vi "Coords.vi"(10 "Data Points":dbl[][](array[numeric])) -> (0 "Reflectivity Vector":dbl[](array[numeric]), 1 "Y Vector":dbl[](array[numeric]), 4 "Z Vector":dbl[](array[numeric]), 5 "X Vector":dbl[](array[numeric]))   [LabVIEW 2017]
panel:
  out "theta":dbl
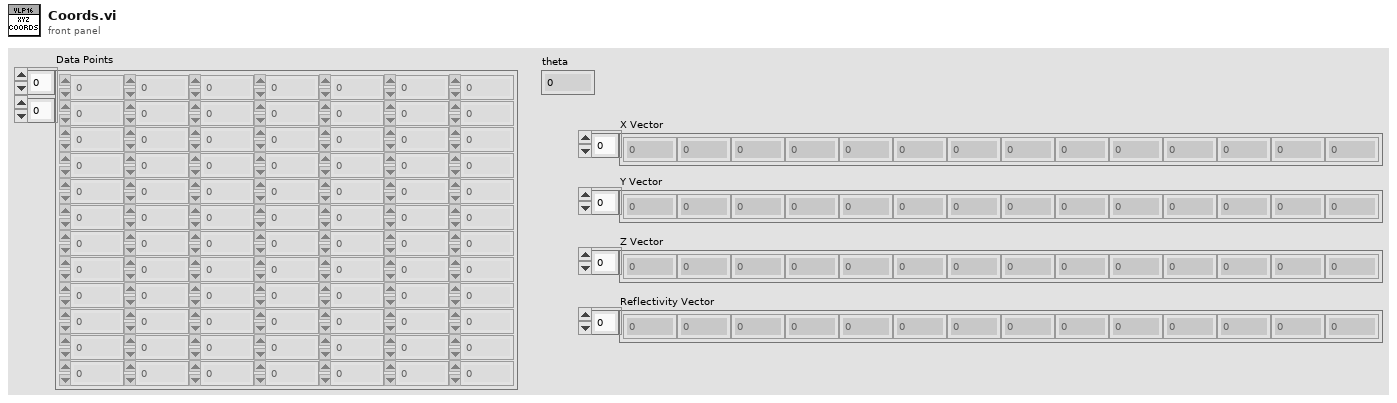
[diagram p1: front panel]
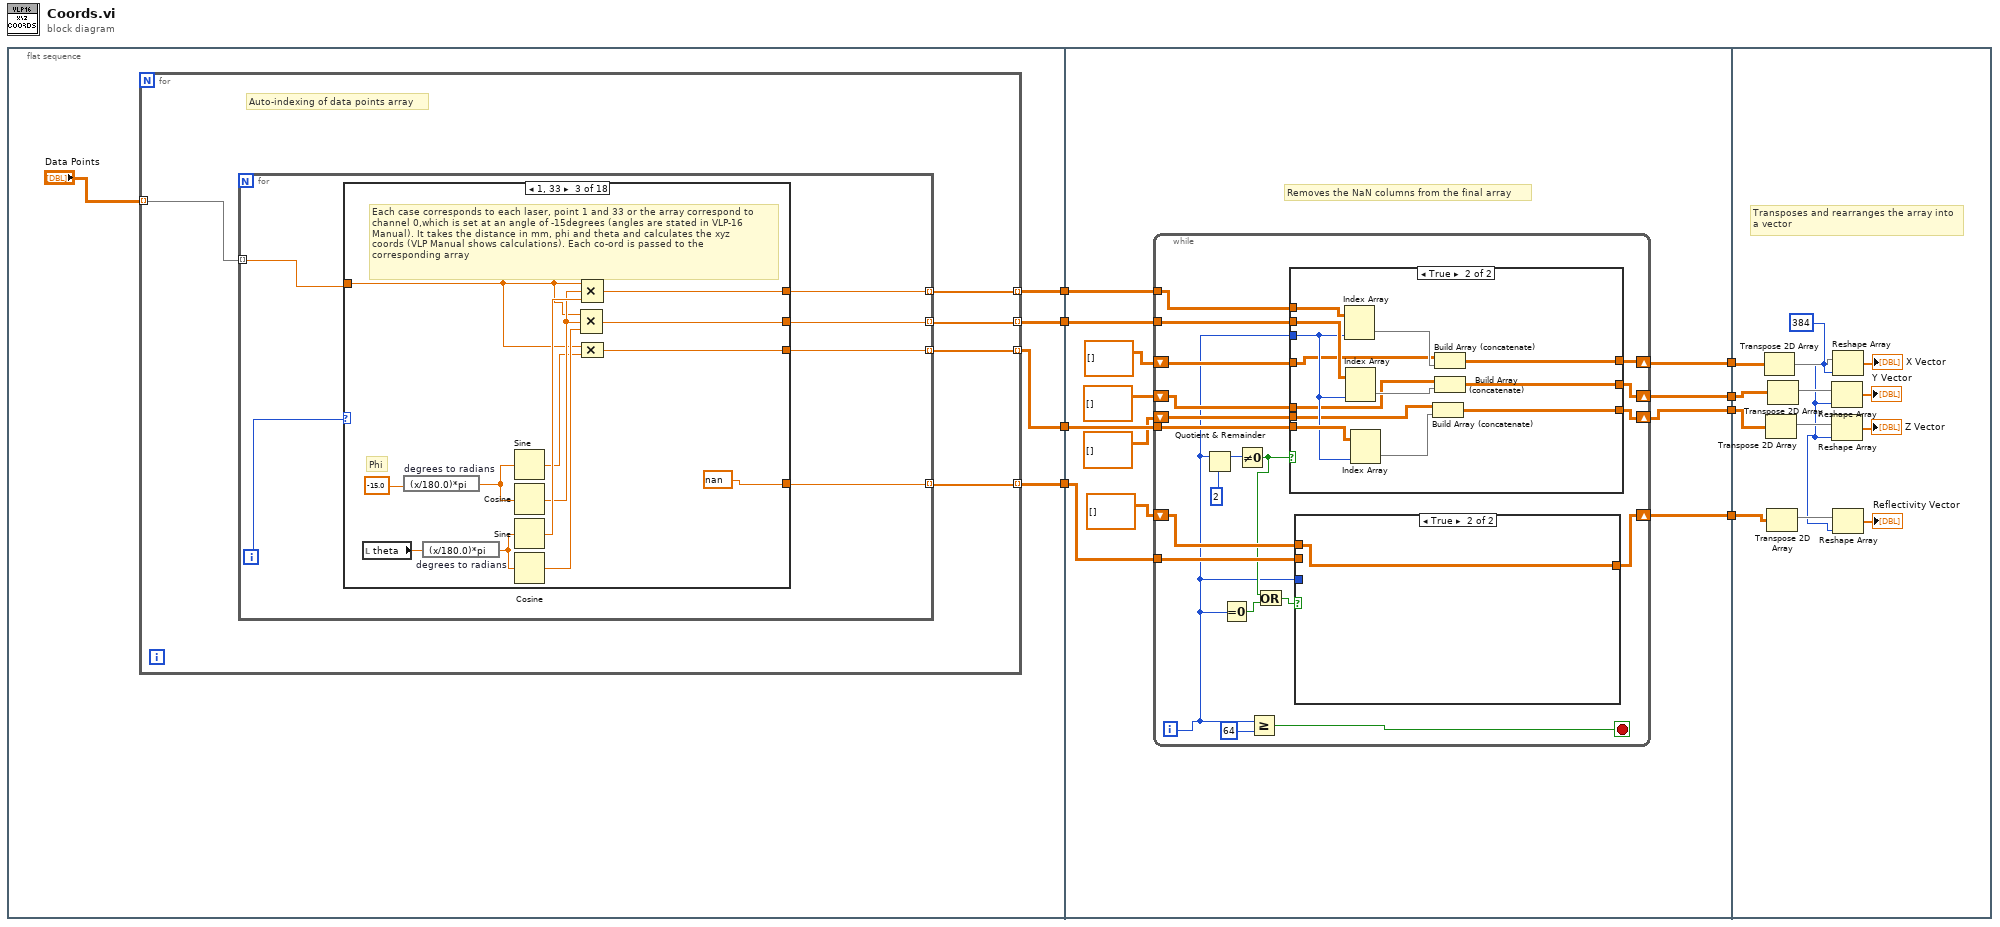
[diagram p0: block diagram]
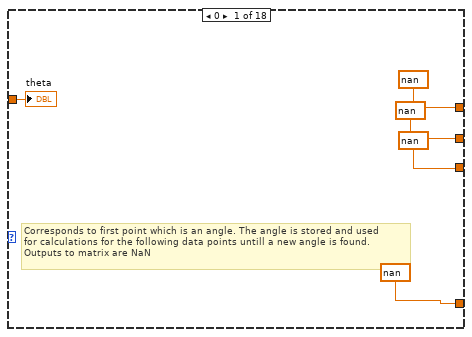
[diagram p2: hidden frame]
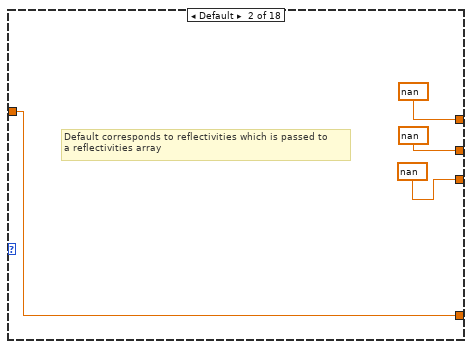
[diagram p3: hidden frame]
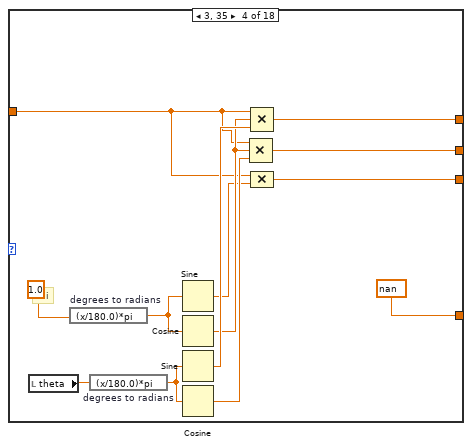
[diagram p4: hidden frame]
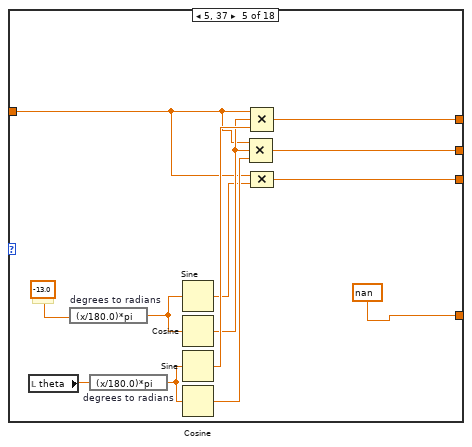
[diagram p5: hidden frame]
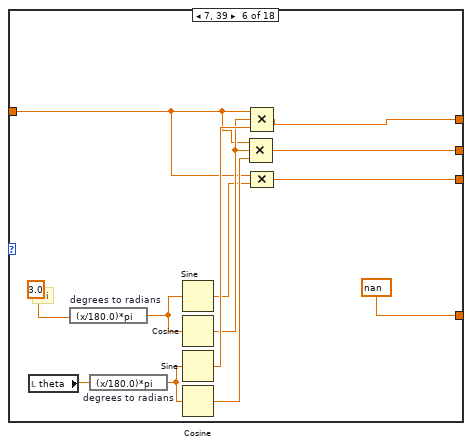
[diagram p6: hidden frame]
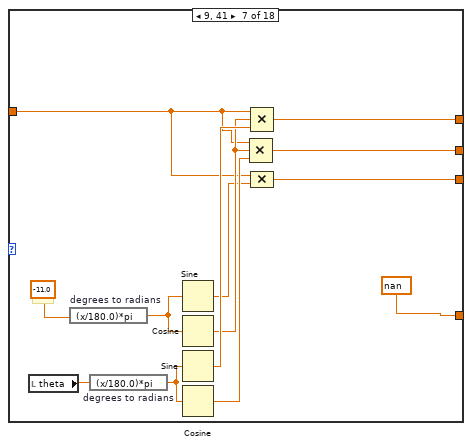
[diagram p7: hidden frame]
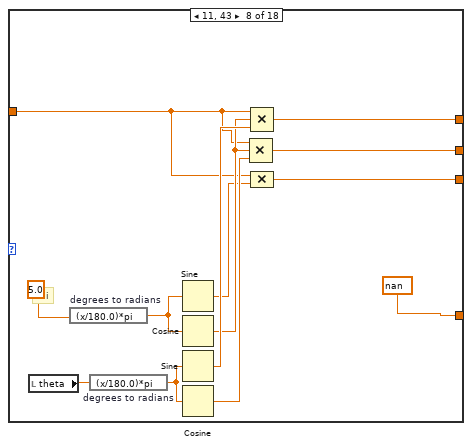
[diagram p8: hidden frame]
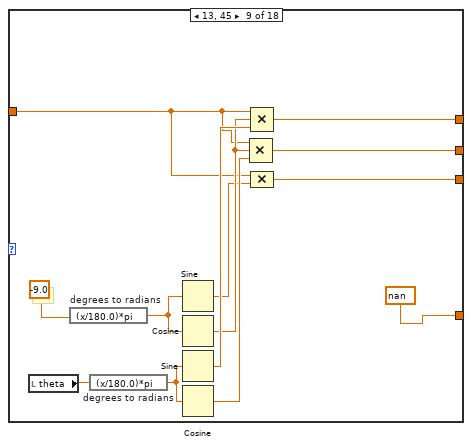
[diagram p9: hidden frame]
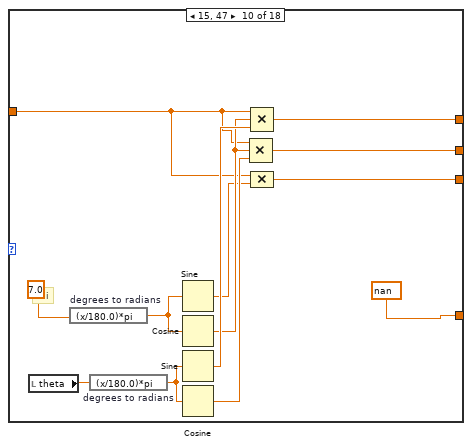
[diagram p10: hidden frame]
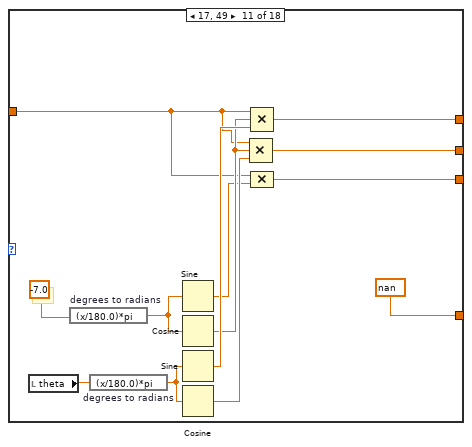
[diagram p11: hidden frame]
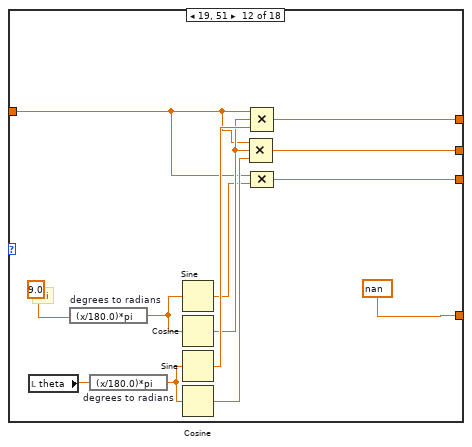
[diagram p12: hidden frame]
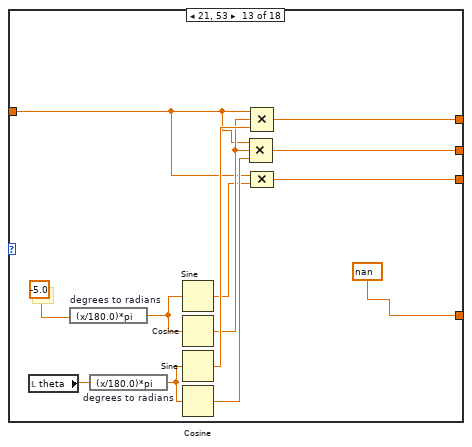
[diagram p13: hidden frame]
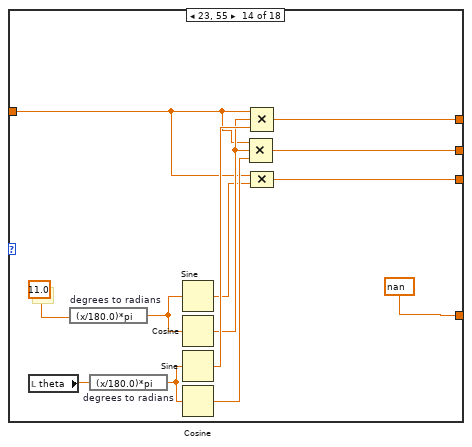
[diagram p14: hidden frame]
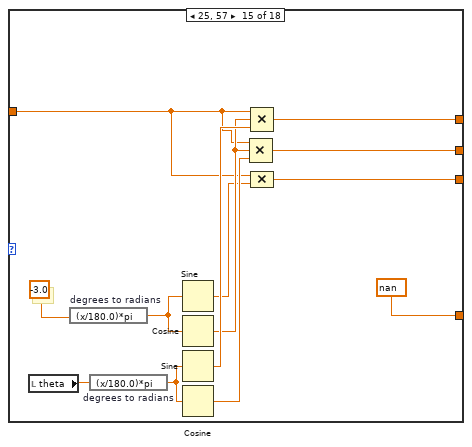
[diagram p15: hidden frame]
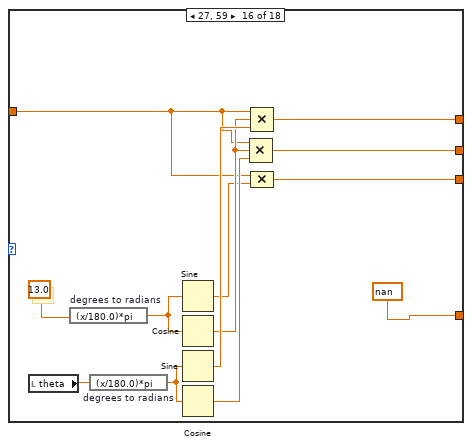
[diagram p16: hidden frame]
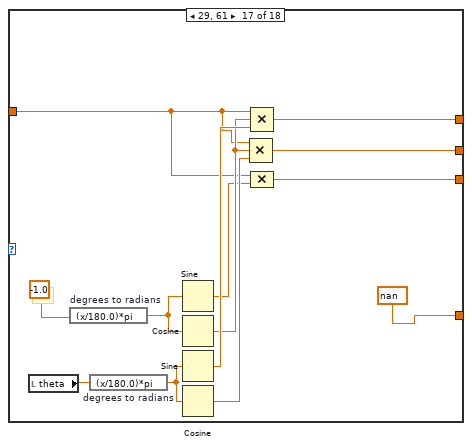
[diagram p17: hidden frame]
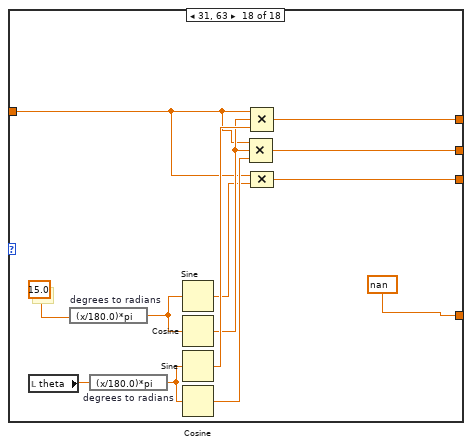
[diagram p18: hidden frame]
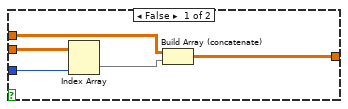
[diagram p19: hidden frame]
diagram:
  n1 = flat-sequence {
    tunnel: [w12] -> w8
    tunnel: [w11] -> w7
    tunnel: [w10] -> w6
    tunnel: [w9] -> w2
    tunnel: w8 -> [w253]
    tunnel: w7 -> [w252]
    tunnel: w6 -> [w251]
    tunnel: [w249] -> w5
    tunnel: [w246] -> w4
    tunnel: [w245] -> w3
    tunnel: w2 -> [w243]
    tunnel: [w242] -> w1
    tunnel: w5 -> [w306]
    tunnel: w4 -> [w307]
    tunnel: w3 -> [w308]
    tunnel: w1 -> [w298]
    frame #0 {
      n2 = for {
        tunnel: "Data Points" -> [w18] mode=indexing
        tunnel: [w17] -> w12 mode=indexing
        tunnel: [w16] -> w11 mode=indexing
        tunnel: [w15] -> w10 mode=indexing
        tunnel: [w14] -> w9 mode=indexing
        # "Auto-indexing of data points array"
        n3 = for {
          tunnel: w18 -> [w23] mode=indexing
          tunnel: [w22] -> w17 mode=indexing
          tunnel: [w21] -> w16 mode=indexing
          tunnel: [w20] -> w15 mode=indexing
          tunnel: [w19] -> w14 mode=indexing
          i -> [w24]
          n4 = case shown="1, 33" w24 {
            tunnel: w23 -> [w29 w30 w43 w56 w69 w82 w95 w108 w121 w134 w147 w160 w173 w186 w199 w212 w225 w238]
            tunnel: [nan nan w37 w50 w63 w76 w89 w102 w115 w128 w141 w154 w167 w180 w193 w206 w219 w232] -> w22
            tunnel: [nan nan w36 w49 w62 w75 w88 w101 w114 w127 w140 w153 w166 w179 w192 w205 w218 w231] -> w21
            tunnel: [nan nan w35 w48 w61 w74 w87 w100 w113 w126 w139 w152 w165 w178 w191 w204 w217 w230] -> w20
            tunnel: [nan w30 nan nan nan nan nan nan nan nan nan nan nan nan nan nan nan nan] -> w19
            frame 0 {
              # "Corresponds to first point which is an angle. The angle is stored and used\nfor calculations for the following data points untill a new angle is found.\nOutputs to matrix are NaN"
              "theta" <- w29
            }
            frame Default {
              # "Default corresponds to reflectivities which is passed to\na reflectivities array"
            }
            frame 1, 33 {
              # "Each case corresponds to each laser, point 1 and 33 or the array correspond to \nchannel 0,which is set at an angle of -15degrees (angles are stated in VLP-16 \nManual). It takes the distance in mm, phi and theta and calculates the xyz \ncoords (VLP Manual shows calculations). Each co-ord is passed to the \ncorresponding array"
              # "Phi"
              n5 = local read "theta"() -> (w38:dbl)
              n6 = expression code="(x/180.0)*pi" "degrees to radians"(-15.0) -> (w40:dbl)
              n7 = expression code="(x/180.0)*pi" "degrees to radians"(w38) -> (w39:dbl)
              n8 = Sine(x=w40) -> (sin(x)=w42:dbl)
              n9 = Cosine(x=w40) -> (cos(x)=w45:dbl)
              n10 = Sine(x=w39) -> (sin(x)=w46:dbl)
              n11 = Cosine(x=w39) -> (cos(x)=w44:dbl)
              n12 = Compound Arithmetic op=MULTIPLY(w43, w45, w44) -> (w36:dbl)
              n13 = Compound Arithmetic op=MULTIPLY(w43, w45, w46) -> (w37:dbl)
              n14 = Compound Arithmetic op=MULTIPLY(w43, w42) -> (w35:dbl)
            }
            frame 3, 35 {
              # "Phi"
              n15 = local read "theta"() -> (w51:dbl)
              n16 = expression code="(x/180.0)*pi" "degrees to radians"(1.0) -> (w53:dbl)
              n17 = expression code="(x/180.0)*pi" "degrees to radians"(w51) -> (w52:dbl)
              n18 = Sine(x=w53) -> (sin(x)=w55:dbl)
              n19 = Cosine(x=w53) -> (cos(x)=w58:dbl)
              n20 = Sine(x=w52) -> (sin(x)=w59:dbl)
              n21 = Cosine(x=w52) -> (cos(x)=w57:dbl)
              n22 = Compound Arithmetic op=MULTIPLY(w56, w58, w57) -> (w49:dbl)
              n23 = Compound Arithmetic op=MULTIPLY(w56, w58, w59) -> (w50:dbl)
              n24 = Compound Arithmetic op=MULTIPLY(w56, w55) -> (w48:dbl)
            }
            frame 5, 37 {
              # "Phi"
              n25 = local read "theta"() -> (w64:dbl)
              n26 = expression code="(x/180.0)*pi" "degrees to radians"(-13.0) -> (w66:dbl)
              n27 = expression code="(x/180.0)*pi" "degrees to radians"(w64) -> (w65:dbl)
              n28 = Sine(x=w66) -> (sin(x)=w68:dbl)
              n29 = Cosine(x=w66) -> (cos(x)=w71:dbl)
              n30 = Sine(x=w65) -> (sin(x)=w72:dbl)
              n31 = Cosine(x=w65) -> (cos(x)=w70:dbl)
              n32 = Compound Arithmetic op=MULTIPLY(w69, w71, w70) -> (w62:dbl)
              n33 = Compound Arithmetic op=MULTIPLY(w69, w71, w72) -> (w63:dbl)
              n34 = Compound Arithmetic op=MULTIPLY(w69, w68) -> (w61:dbl)
            }
            frame 7, 39 {
              # "Phi"
              n35 = local read "theta"() -> (w77:dbl)
              n36 = expression code="(x/180.0)*pi" "degrees to radians"(3.0) -> (w79:dbl)
              n37 = expression code="(x/180.0)*pi" "degrees to radians"(w77) -> (w78:dbl)
              n38 = Sine(x=w79) -> (sin(x)=w81:dbl)
              n39 = Cosine(x=w79) -> (cos(x)=w84:dbl)
              n40 = Sine(x=w78) -> (sin(x)=w85:dbl)
              n41 = Cosine(x=w78) -> (cos(x)=w83:dbl)
              n42 = Compound Arithmetic op=MULTIPLY(w82, w84, w83) -> (w75:dbl)
              n43 = Compound Arithmetic op=MULTIPLY(w82, w84, w85) -> (w76:dbl)
              n44 = Compound Arithmetic op=MULTIPLY(w82, w81) -> (w74:dbl)
            }
            frame 9, 41 {
              # "Phi"
              n45 = local read "theta"() -> (w90:dbl)
              n46 = expression code="(x/180.0)*pi" "degrees to radians"(-11.0) -> (w92:dbl)
              n47 = expression code="(x/180.0)*pi" "degrees to radians"(w90) -> (w91:dbl)
              n48 = Sine(x=w92) -> (sin(x)=w94:dbl)
              n49 = Cosine(x=w92) -> (cos(x)=w97:dbl)
              n50 = Sine(x=w91) -> (sin(x)=w98:dbl)
              n51 = Cosine(x=w91) -> (cos(x)=w96:dbl)
              n52 = Compound Arithmetic op=MULTIPLY(w95, w97, w96) -> (w88:dbl)
              n53 = Compound Arithmetic op=MULTIPLY(w95, w97, w98) -> (w89:dbl)
              n54 = Compound Arithmetic op=MULTIPLY(w95, w94) -> (w87:dbl)
            }
            frame 11, 43 {
              # "Phi"
              n55 = local read "theta"() -> (w103:dbl)
              n56 = expression code="(x/180.0)*pi" "degrees to radians"(5.0) -> (w105:dbl)
              n57 = expression code="(x/180.0)*pi" "degrees to radians"(w103) -> (w104:dbl)
              n58 = Sine(x=w105) -> (sin(x)=w107:dbl)
              n59 = Cosine(x=w105) -> (cos(x)=w110:dbl)
              n60 = Sine(x=w104) -> (sin(x)=w111:dbl)
              n61 = Cosine(x=w104) -> (cos(x)=w109:dbl)
              n62 = Compound Arithmetic op=MULTIPLY(w108, w110, w109) -> (w101:dbl)
              n63 = Compound Arithmetic op=MULTIPLY(w108, w110, w111) -> (w102:dbl)
              n64 = Compound Arithmetic op=MULTIPLY(w108, w107) -> (w100:dbl)
            }
            frame 13, 45 {
              # "Phi"
              n65 = local read "theta"() -> (w116:dbl)
              n66 = expression code="(x/180.0)*pi" "degrees to radians"(-9.0) -> (w118:dbl)
              n67 = expression code="(x/180.0)*pi" "degrees to radians"(w116) -> (w117:dbl)
              n68 = Sine(x=w118) -> (sin(x)=w120:dbl)
              n69 = Cosine(x=w118) -> (cos(x)=w123:dbl)
              n70 = Sine(x=w117) -> (sin(x)=w124:dbl)
              n71 = Cosine(x=w117) -> (cos(x)=w122:dbl)
              n72 = Compound Arithmetic op=MULTIPLY(w121, w123, w122) -> (w114:dbl)
              n73 = Compound Arithmetic op=MULTIPLY(w121, w123, w124) -> (w115:dbl)
              n74 = Compound Arithmetic op=MULTIPLY(w121, w120) -> (w113:dbl)
            }
            frame 15, 47 {
              # "Phi"
              n75 = local read "theta"() -> (w129:dbl)
              n76 = expression code="(x/180.0)*pi" "degrees to radians"(7.0) -> (w131:dbl)
              n77 = expression code="(x/180.0)*pi" "degrees to radians"(w129) -> (w130:dbl)
              n78 = Sine(x=w131) -> (sin(x)=w133:dbl)
              n79 = Cosine(x=w131) -> (cos(x)=w136:dbl)
              n80 = Sine(x=w130) -> (sin(x)=w137:dbl)
              n81 = Cosine(x=w130) -> (cos(x)=w135:dbl)
              n82 = Compound Arithmetic op=MULTIPLY(w134, w136, w135) -> (w127:dbl)
              n83 = Compound Arithmetic op=MULTIPLY(w134, w136, w137) -> (w128:dbl)
              n84 = Compound Arithmetic op=MULTIPLY(w134, w133) -> (w126:dbl)
            }
            frame 17, 49 {
              # "Phi"
              n85 = local read "theta"() -> (w142:dbl)
              n86 = expression code="(x/180.0)*pi" "degrees to radians"(-7.0) -> (w144:dbl)
              n87 = expression code="(x/180.0)*pi" "degrees to radians"(w142) -> (w143:dbl)
              n88 = Sine(x=w144) -> (sin(x)=w146:dbl)
              n89 = Cosine(x=w144) -> (cos(x)=w149:dbl)
              n90 = Sine(x=w143) -> (sin(x)=w150:dbl)
              n91 = Cosine(x=w143) -> (cos(x)=w148:dbl)
              n92 = Compound Arithmetic op=MULTIPLY(w147, w149, w148) -> (w140:dbl)
              n93 = Compound Arithmetic op=MULTIPLY(w147, w149, w150) -> (w141:dbl)
              n94 = Compound Arithmetic op=MULTIPLY(w147, w146) -> (w139:dbl)
            }
            frame 19, 51 {
              # "Phi"
              n95 = local read "theta"() -> (w155:dbl)
              n96 = expression code="(x/180.0)*pi" "degrees to radians"(9.0) -> (w157:dbl)
              n97 = expression code="(x/180.0)*pi" "degrees to radians"(w155) -> (w156:dbl)
              n98 = Sine(x=w157) -> (sin(x)=w159:dbl)
              n99 = Cosine(x=w157) -> (cos(x)=w162:dbl)
              n100 = Sine(x=w156) -> (sin(x)=w163:dbl)
              n101 = Cosine(x=w156) -> (cos(x)=w161:dbl)
              n102 = Compound Arithmetic op=MULTIPLY(w160, w162, w161) -> (w153:dbl)
              n103 = Compound Arithmetic op=MULTIPLY(w160, w162, w163) -> (w154:dbl)
              n104 = Compound Arithmetic op=MULTIPLY(w160, w159) -> (w152:dbl)
            }
            frame 21, 53 {
              # "Phi"
              n105 = local read "theta"() -> (w168:dbl)
              n106 = expression code="(x/180.0)*pi" "degrees to radians"(-5.0) -> (w170:dbl)
              n107 = expression code="(x/180.0)*pi" "degrees to radians"(w168) -> (w169:dbl)
              n108 = Sine(x=w170) -> (sin(x)=w172:dbl)
              n109 = Cosine(x=w170) -> (cos(x)=w175:dbl)
              n110 = Sine(x=w169) -> (sin(x)=w176:dbl)
              n111 = Cosine(x=w169) -> (cos(x)=w174:dbl)
              n112 = Compound Arithmetic op=MULTIPLY(w173, w175, w174) -> (w166:dbl)
              n113 = Compound Arithmetic op=MULTIPLY(w173, w175, w176) -> (w167:dbl)
              n114 = Compound Arithmetic op=MULTIPLY(w173, w172) -> (w165:dbl)
            }
            frame 23, 55 {
              # "Phi"
              n115 = local read "theta"() -> (w181:dbl)
              n116 = expression code="(x/180.0)*pi" "degrees to radians"(11.0) -> (w183:dbl)
              n117 = expression code="(x/180.0)*pi" "degrees to radians"(w181) -> (w182:dbl)
              n118 = Sine(x=w183) -> (sin(x)=w185:dbl)
              n119 = Cosine(x=w183) -> (cos(x)=w188:dbl)
              n120 = Sine(x=w182) -> (sin(x)=w189:dbl)
              n121 = Cosine(x=w182) -> (cos(x)=w187:dbl)
              n122 = Compound Arithmetic op=MULTIPLY(w186, w188, w187) -> (w179:dbl)
              n123 = Compound Arithmetic op=MULTIPLY(w186, w188, w189) -> (w180:dbl)
              n124 = Compound Arithmetic op=MULTIPLY(w186, w185) -> (w178:dbl)
            }
            frame 25, 57 {
              # "Phi"
              n125 = local read "theta"() -> (w194:dbl)
              n126 = expression code="(x/180.0)*pi" "degrees to radians"(-3.0) -> (w196:dbl)
              n127 = expression code="(x/180.0)*pi" "degrees to radians"(w194) -> (w195:dbl)
              n128 = Sine(x=w196) -> (sin(x)=w198:dbl)
              n129 = Cosine(x=w196) -> (cos(x)=w201:dbl)
              n130 = Sine(x=w195) -> (sin(x)=w202:dbl)
              n131 = Cosine(x=w195) -> (cos(x)=w200:dbl)
              n132 = Compound Arithmetic op=MULTIPLY(w199, w201, w200) -> (w192:dbl)
              n133 = Compound Arithmetic op=MULTIPLY(w199, w201, w202) -> (w193:dbl)
              n134 = Compound Arithmetic op=MULTIPLY(w199, w198) -> (w191:dbl)
            }
            frame 27, 59 {
              # "Phi"
              n135 = local read "theta"() -> (w207:dbl)
              n136 = expression code="(x/180.0)*pi" "degrees to radians"(13.0) -> (w209:dbl)
              n137 = expression code="(x/180.0)*pi" "degrees to radians"(w207) -> (w208:dbl)
              n138 = Sine(x=w209) -> (sin(x)=w211:dbl)
              n139 = Cosine(x=w209) -> (cos(x)=w214:dbl)
              n140 = Sine(x=w208) -> (sin(x)=w215:dbl)
              n141 = Cosine(x=w208) -> (cos(x)=w213:dbl)
              n142 = Compound Arithmetic op=MULTIPLY(w212, w214, w213) -> (w205:dbl)
              n143 = Compound Arithmetic op=MULTIPLY(w212, w214, w215) -> (w206:dbl)
              n144 = Compound Arithmetic op=MULTIPLY(w212, w211) -> (w204:dbl)
            }
            frame 29, 61 {
              # "Phi"
              n145 = local read "theta"() -> (w220:dbl)
              n146 = expression code="(x/180.0)*pi" "degrees to radians"(-1.0) -> (w222:dbl)
              n147 = expression code="(x/180.0)*pi" "degrees to radians"(w220) -> (w221:dbl)
              n148 = Sine(x=w222) -> (sin(x)=w224:dbl)
              n149 = Cosine(x=w222) -> (cos(x)=w227:dbl)
              n150 = Sine(x=w221) -> (sin(x)=w228:dbl)
              n151 = Cosine(x=w221) -> (cos(x)=w226:dbl)
              n152 = Compound Arithmetic op=MULTIPLY(w225, w227, w226) -> (w218:dbl)
              n153 = Compound Arithmetic op=MULTIPLY(w225, w227, w228) -> (w219:dbl)
              n154 = Compound Arithmetic op=MULTIPLY(w225, w224) -> (w217:dbl)
            }
            frame 31, 63 {
              # "Phi"
              n155 = local read "theta"() -> (w233:dbl)
              n156 = expression code="(x/180.0)*pi" "degrees to radians"(15.0) -> (w235:dbl)
              n157 = expression code="(x/180.0)*pi" "degrees to radians"(w233) -> (w234:dbl)
              n158 = Sine(x=w235) -> (sin(x)=w237:dbl)
              n159 = Cosine(x=w235) -> (cos(x)=w240:dbl)
              n160 = Sine(x=w234) -> (sin(x)=w241:dbl)
              n161 = Cosine(x=w234) -> (cos(x)=w239:dbl)
              n162 = Compound Arithmetic op=MULTIPLY(w238, w240, w239) -> (w231:dbl)
              n163 = Compound Arithmetic op=MULTIPLY(w238, w240, w241) -> (w232:dbl)
              n164 = Compound Arithmetic op=MULTIPLY(w238, w237) -> (w230:dbl)
            }
          }
        }
      }
    }
    frame #1 {
      # "Removes the NaN columns from the final array"
      n165 = while {
        tunnel: w253 -> [w269]
        tunnel: w252 -> [w268]
        tunnel: w251 -> [w267]
        shift-right: [w264] -> w249
        shift-left: dbl[][] [] -> [w265]
        shift-right: [w263] -> w246
        shift-left: dbl[][] [] -> [w266]
        shift-right: [w261] -> w245
        shift-left: dbl[][] [] -> [w262]
        shift-right: [w258] -> w242
        shift-left: dbl[][] [] -> [w259]
        tunnel: w243 -> [w260]
        i -> [w256]
        stop <- w272 stop-if-true
        n166 = Quotient & Remainder(x=w256, y=2) -> (x-y*floor(x/y)=w270:i32)  [unwired: 1 out]
        n167 = Equal To 0?(x=w256) -> (x = 0?=w255:bool)
        n168 = Not Equal To 0?(x=w270) -> (x != 0?=w257:bool)
        n169 = Greater Or Equal?(x=w256, y=64) -> (x >= y?=w272:bool)
        n170 = Or(x=w257, y=w255) -> (x .or. y?=w254:bool)
        n171 = case shown="True" w257 {
          tunnel: w269 -> [_ w295]
          tunnel: w256 -> [_ w292]
          tunnel: w268 -> [_ w294]
          tunnel: w266 -> [w281 w285]
          tunnel: w267 -> [_ w293]
          tunnel: w265 -> [w280 w283]
          tunnel: [w282 w291] -> w261
          tunnel: [w281 w290] -> w263
          tunnel: [w280 w289] -> w264
          tunnel: w262 -> [w282 w287]
          frame False {
          }
          frame True {
            n172 = Index Array(array=w295, index (col)=w292) -> (element=w288:dbl[])  [unwired: 1 in]
            n173 = Index Array(array=w294, index (col)=w292) -> (element=w286:dbl[])  [unwired: 1 in]
            n174 = Index Array(array=w293, index (col)=w292) -> (element=w284:dbl[])  [unwired: 1 in]
            n175 = Build Array (concatenate)(w283, w284) -> (w289:dbl[][])
            n176 = Build Array (concatenate)(w287, w288) -> (w291:dbl[][])
            n177 = Build Array (concatenate)(w285, w286) -> (w290:dbl[][])
          }
        }
        n178 = case shown="True" w254 {
          tunnel: w260 -> [w278 _]
          tunnel: w256 -> [w277 _]
          tunnel: w259 -> [w276 w279]
          tunnel: [w274 w279] -> w258
          frame False {
            n179 = Index Array(array=w278, index (col)=w277) -> (element=w275:dbl[])  [unwired: 1 in]
            n180 = Build Array (concatenate)(w276, w275) -> (w274:dbl[][])
          }
          frame True {
          }
        }
      }
    }
    frame #2 {
      w297 = 384 ("dimension size")
      # "Transposes and rearranges the array into\na vector"
      n181 = Transpose 2D Array(2D array=w308) -> (transposed array=w305:dbl[][])
      n182 = Transpose 2D Array(2D array=w306) -> (transposed array=w303:dbl[][])
      n183 = Transpose 2D Array(2D array=w298) -> (transposed array=w299:dbl[][])
      n184 = Transpose 2D Array(2D array=w307) -> (transposed array=w304:dbl[][])
      n185 = Reshape Array(w304, w297) -> (→"Y Vector":dbl[])
      n186 = Reshape Array(w303, w297) -> (→"Z Vector":dbl[])
      n187 = Reshape Array(w305, w297) -> (→"X Vector":dbl[])
      n188 = Reshape Array(w299, w297) -> (→"Reflectivity Vector":dbl[])
    }
  }
